vi "Close (SubVI).vi"(2 "DeviceKey Out":string, 8 "error in":errorcluster, 11 "CmdLib In":refnum<k24>) -> (0 "error out":errorcluster, 3 "CmdLib Out":refnum<k24>)   [LabVIEW 2017]
uses:
  dll/CmdLib.dll
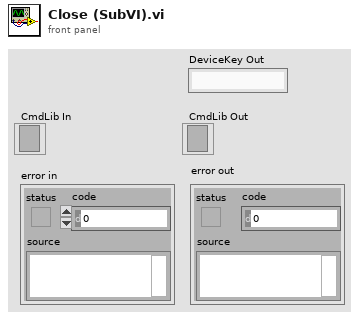
[diagram p1: front panel]
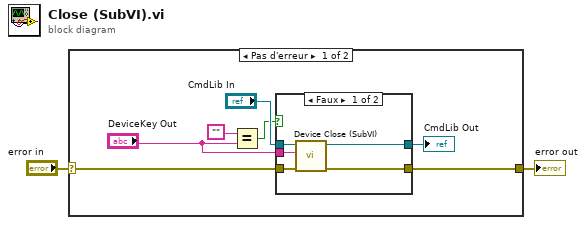
[diagram p0: block diagram]
diagram:
  n1 = case shown="Pas d'erreur" "error in" {
    selector: "error in" -> [w4 w17]
    tunnel: [w8 w17] -> w2
    frame No Error {
      n2 = Equal?(x="", y="DeviceKey Out") -> (x = y?=w5:bool)
      n3 = case shown="Faux" w5 {
        tunnel: [w14 w16] -> w7
        tunnel: [w13 w15] -> w8
        tunnel: w4 -> [w12 w15]
        tunnel: "CmdLib In" -> [w11 w16]
        tunnel: "DeviceKey Out" -> [w10 _]
        frame False {
          n4 = call "Device Close (SubVI).vi"("error in (no error)"=w12, "DeviceKey In"=w10, "CmdLib In"=w11) -> ("error out"=w13:errorcluster, "CmdLib Out"=w14:refnum<k24>)  [unwired: 6 in, 1 out]
        }
        frame True {
        }
      }
      "CmdLib Out" <- w7
    }
    frame Error {
    }
  }
  "error out" <- w2
